vi "Setting.vi"() -> ()   [LabVIEW 2015]
uses:
  enum/Control_PanelControl.ctl
  enum/Control_FileControl.ctl
  enum/Control_ExitControl.ctl
  enum/Control_IOControl.ctl
  enum/Control_CameraControl.ctl
  enum/Control_ImageControl.ctl
  enum/Control_Inspection.ctl
  enum/Control_InspectionItem.ctl
  enum/Control_ErrorControl.ctl
  enum/Control_IdleControl.ctl
  enum/Control_MachineVerification.ctl
  enum/Control_DialogControl.ctl
  enum/Control_LightControl.ctl
  <vilib>/Utility/miscctls.llb/LVPointTypeDef.ctl
  <userlib>/FGV/control/Control_Indicator Action.ctl
  <userlib>/FGV/control/Control_Image.ctl
  <userlib>/FGV/control/Control_Camera.ctl
  <userlib>/FGV/control/Control_Data.ctl
  <vilib>/userdefined/High Color/IMAQdx.ctl
panel:
  in  "start path":path=path "D:/渦輪組裝機參數/Data 資料/Setting Data"
  in  "file (use dialog)":path=path "D:/渦輪組裝機參數/Data 資料/Setting Data"
  out "Image":T1(plugin-control)
  in  "匯入圖片":bool
  out "input cluster":T2
  in  "Control":T3
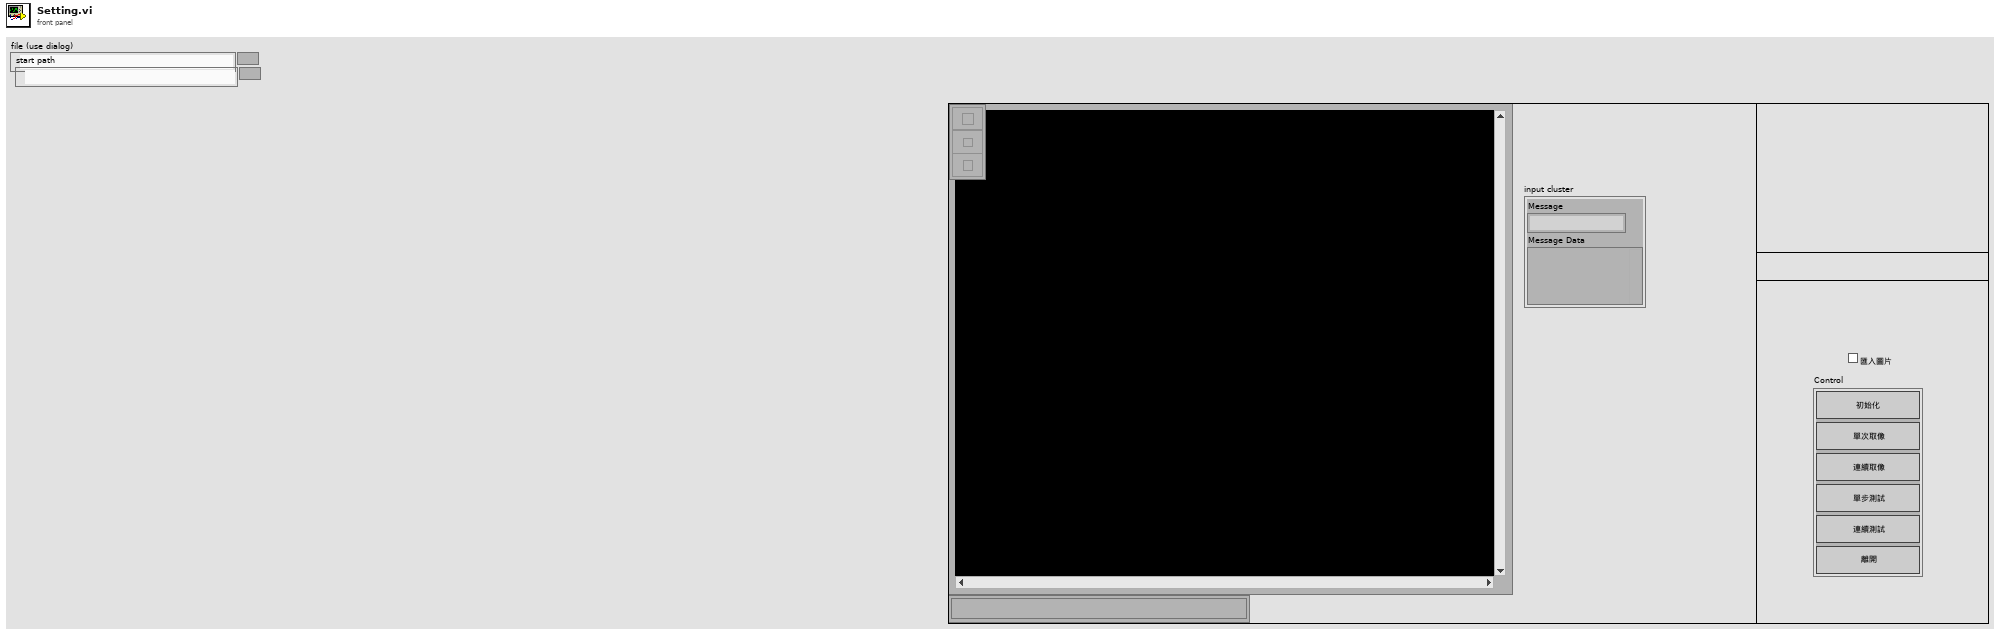
[diagram p1: front panel]
types:
  T1 = typedef "IMAQ Image.ctl" = refnum<image>
  T2 = cluster{"Message":string, "Message Data":variant}
  T3 = cluster{"一、動作-初始化":bool, "二、動作-單次取像":bool, "三、動作-連續取像":bool, "四、動作-單步測試":bool, "五、動作-連續測試":bool, "六、動作-離開":bool}
  T4 = typedef "LVPointTypeDef.ctl" = cluster{"Horizontal":i16, "Vertical":i16}
  T5 = typedef "Control_LightControl.ctl" = enum16{"1.光源控制-初始化", "2.光源控制-光源開啟", "3.光源控制-光源關閉", "4.光源控制-通訊關閉"}
  T6 = typedef "Control_DialogControl.ctl" = enum16{"1.對話視窗"}
  T7 = typedef "Control_MachineVerification.ctl" = enum16{"1.機台驗證-初始化", "2.機台驗證-檢測"}
  T8 = typedef "Control_ExitControl.ctl" = enum16{"1.離開"}
  T9 = typedef "Control_IdleControl.ctl" = enum16{"1.等待(計算時間)"}
  T10 = typedef "Control_ErrorControl.ctl" = enum16{"1.錯誤"}
  T11 = typedef "Control_FileControl.ctl" = enum16{"1.檔案-初始化", "2.檔案-儲存檔案", "3.檔案-開啟檔案", "4.檔案-匯入檔案"}
  T12 = typedef "Control_InspectionItem.ctl" = enum16{"FindPositionXY", "Match"}
  T13 = typedef "Control_Inspection.ctl" = enum16{"1.檢測-初始化", "2.浪代-浪代"}
  T14 = typedef "Control_ImageControl.ctl" = enum16{"1.影像-初始化", "2.影像-更新影像", "3.影像-儲存影像"}
  T15 = typedef "Control_CameraControl.ctl" = enum16{"1.相機-初始化", "2.相機-取像", "3.相機-關閉"}
  T16 = typedef "Control_IOControl.ctl" = enum16{"1.IO-初始化", "2. Set Point(EOT On)", "3.Set Point(EOT Off)", "4.Get Point(SOT)"}
  T17 = typedef "Control_PanelControl.ctl" = enum16{"一、動作-初始化", "二、動作-單次取像", "三、動作-連續取像", "四、動作-單步測試", "五、動作-連續測試", "六、動作-離開"}
  T18 = enum16{"一、動作-初始化", "二、動作-單次取像", "三、動作-連續取像", "四、動作-單步測試", "五、動作-連續測試", "六、動作-離開"}
  T19 = typedef "IMAQdx.ctl" = refnum<k21>
  T20 = typedef "Control_Camera.ctl" = enum16{"初始化", "取像", "匯入影像", "結束"}
  T21 = typedef "Control_Image.ctl" = enum16{"初始化", "創造記憶體", "寫入圖片", "讀取圖片", "刪除圖片", "等待"}
  T22 = typedef "Control_Indicator Action.ctl" = enum16{"Set Data", "Get Data", "Idle"}
  T23 = typedef "Control_Data.ctl" = enum16{"Initialize", "Get Data", "Set Data", "Delete Data", "Idle"}
  T24 = cluster{"Message":string, "Message Data":variant}[]
  T25 = cluster{"Label.Text":string, "Variant":variant}[]
  T26 = typedef "Control_Indicator.ctl" = cluster{"相機、光源":cluster{"相機選擇":u8, "光源選擇":u16, "光源亮度":u8}, "Session Out":T19, "Cam#Light#Strength":string}
  T27 = typedef "Image Type" = u32
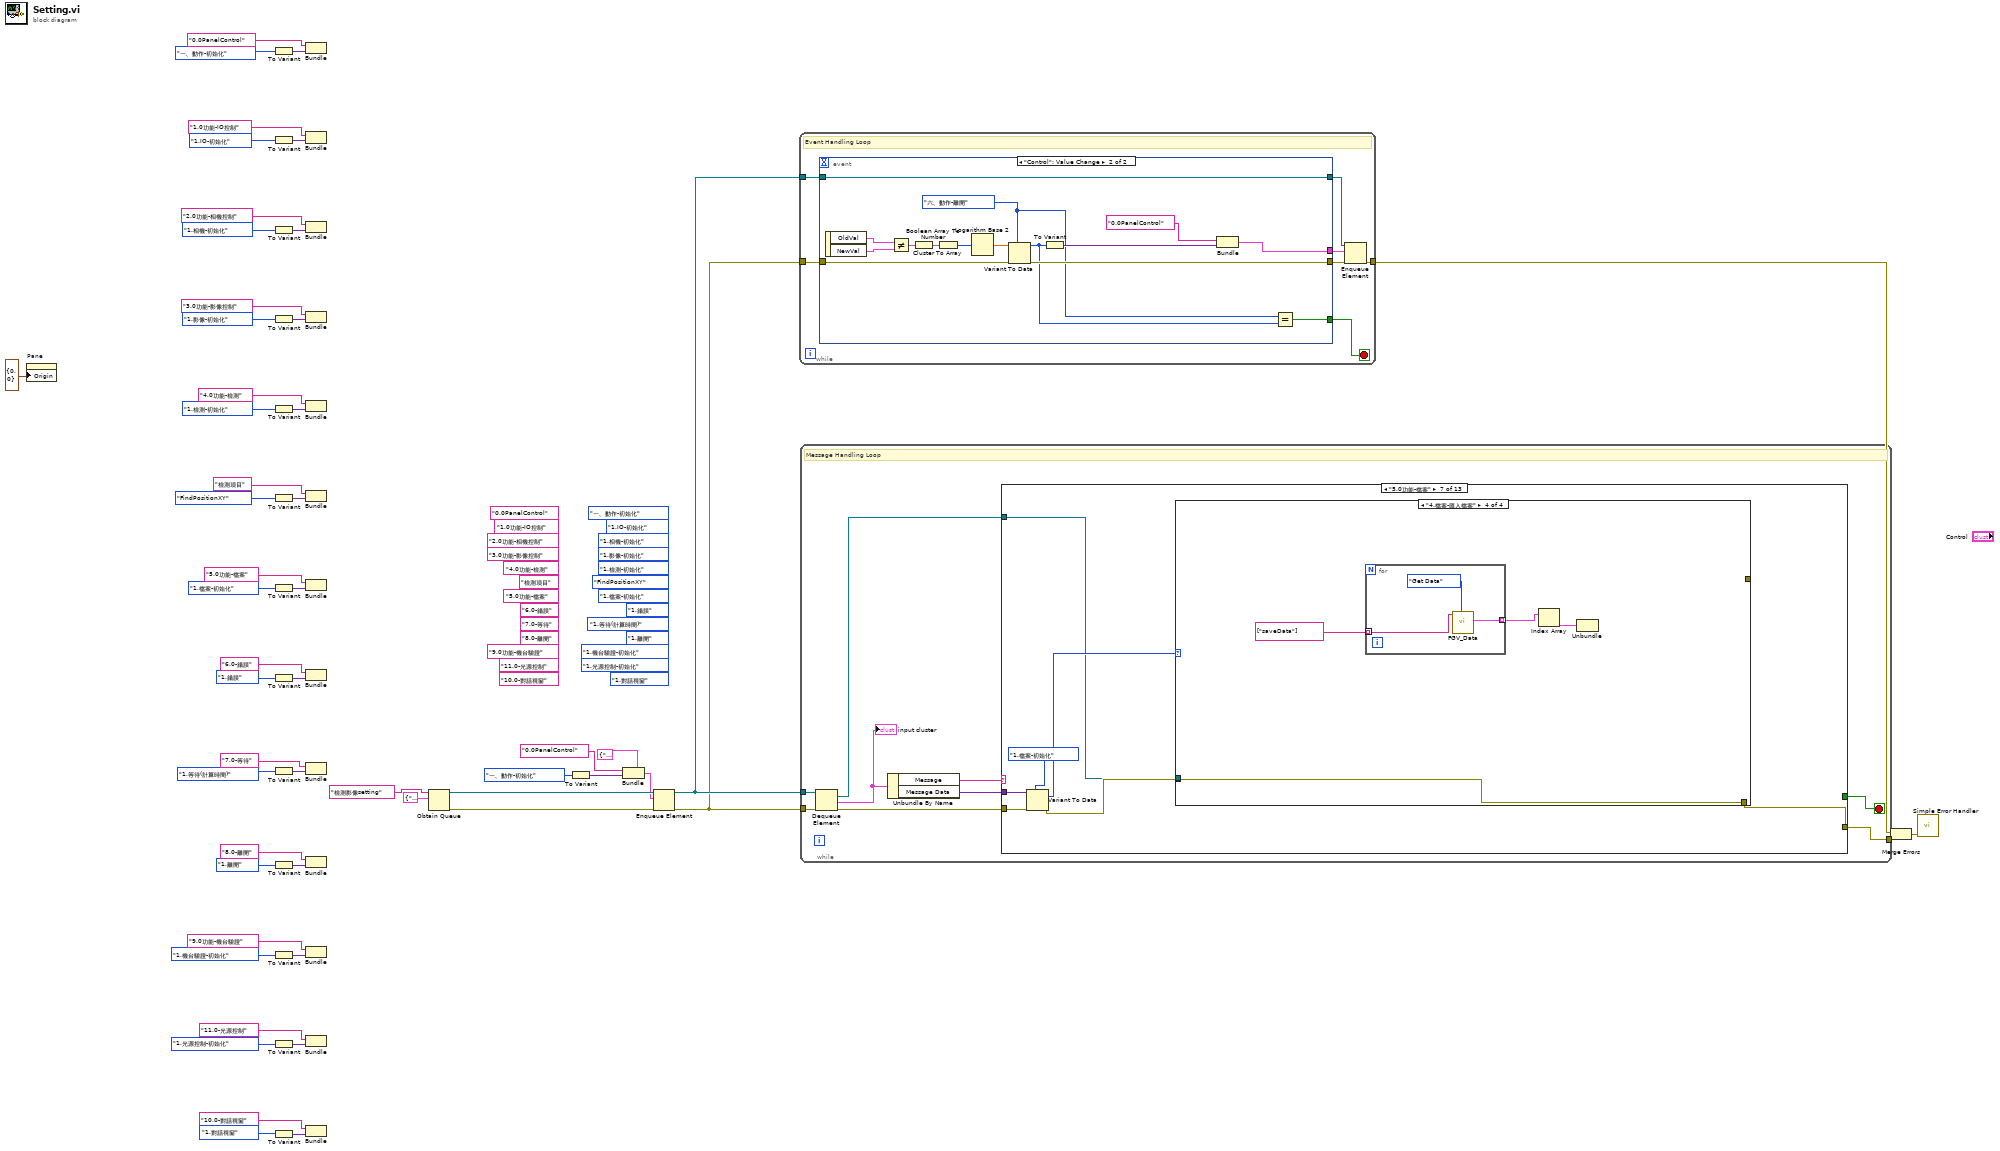
[diagram p0: block diagram]
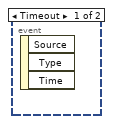
[diagram p2: hidden frame]
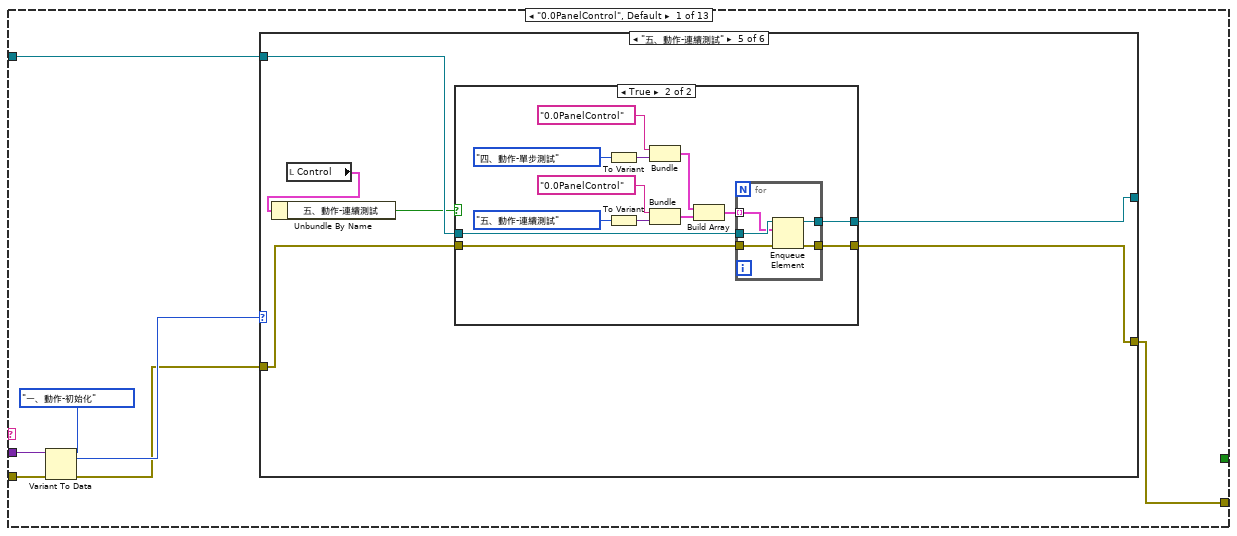
[diagram p3: hidden frame]
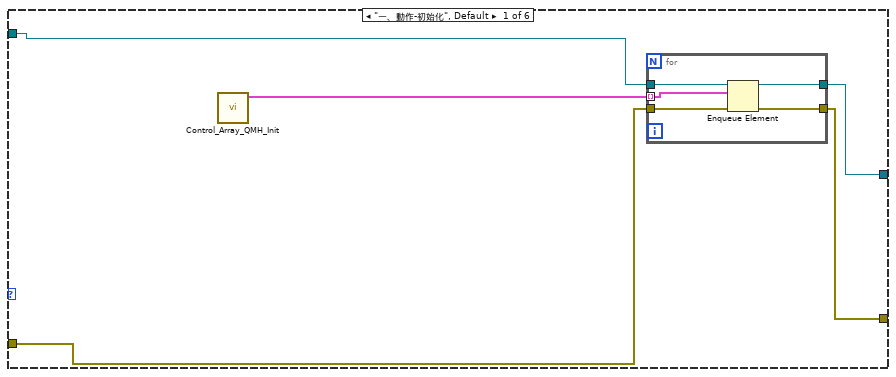
[diagram p4: hidden frame]
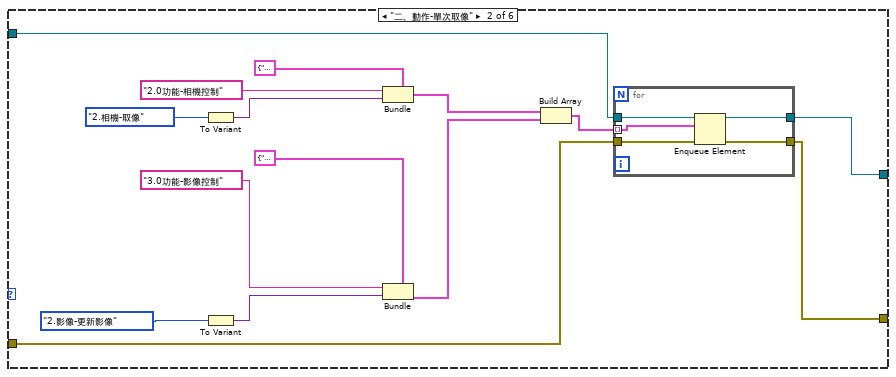
[diagram p5: hidden frame]
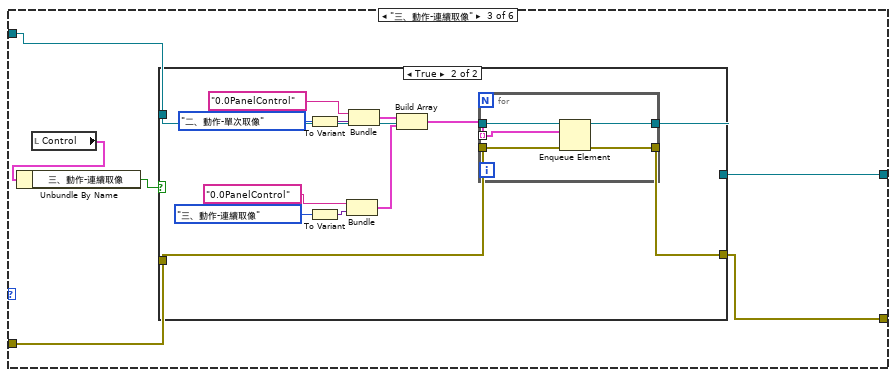
[diagram p6: hidden frame]
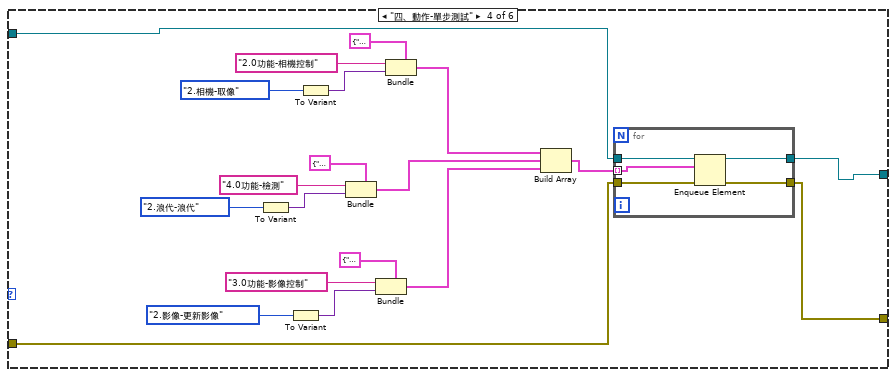
[diagram p8: hidden frame]
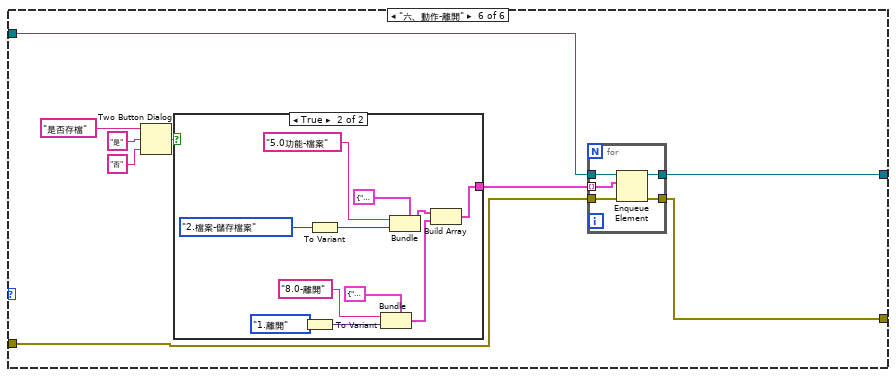
[diagram p10: hidden frame]
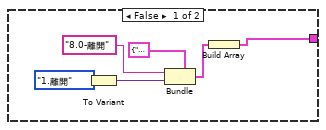
[diagram p11: hidden frame]
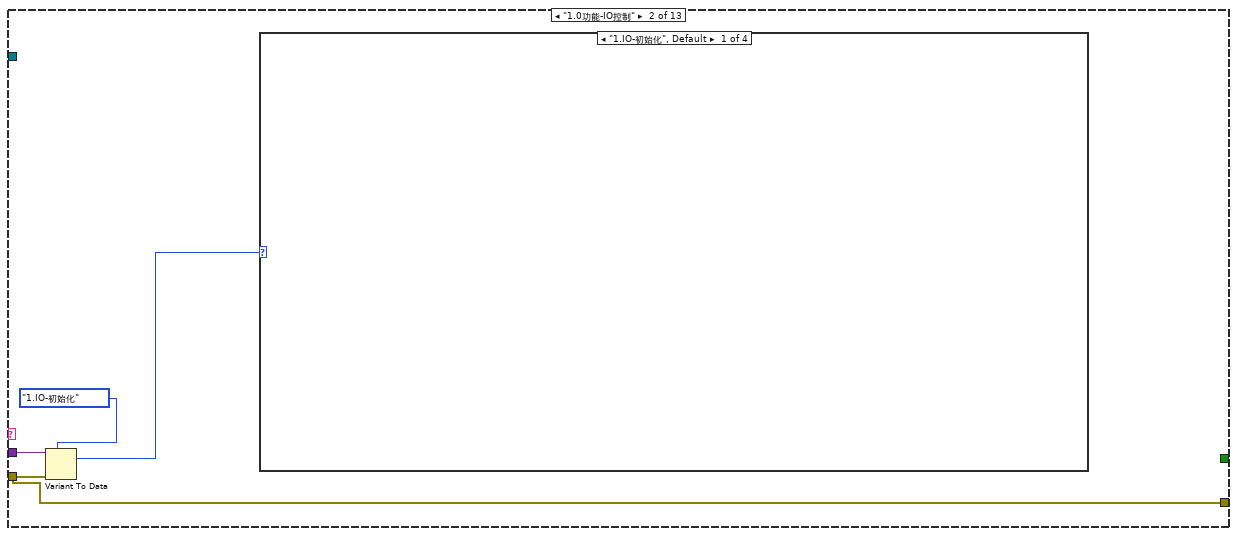
[diagram p12: hidden frame]
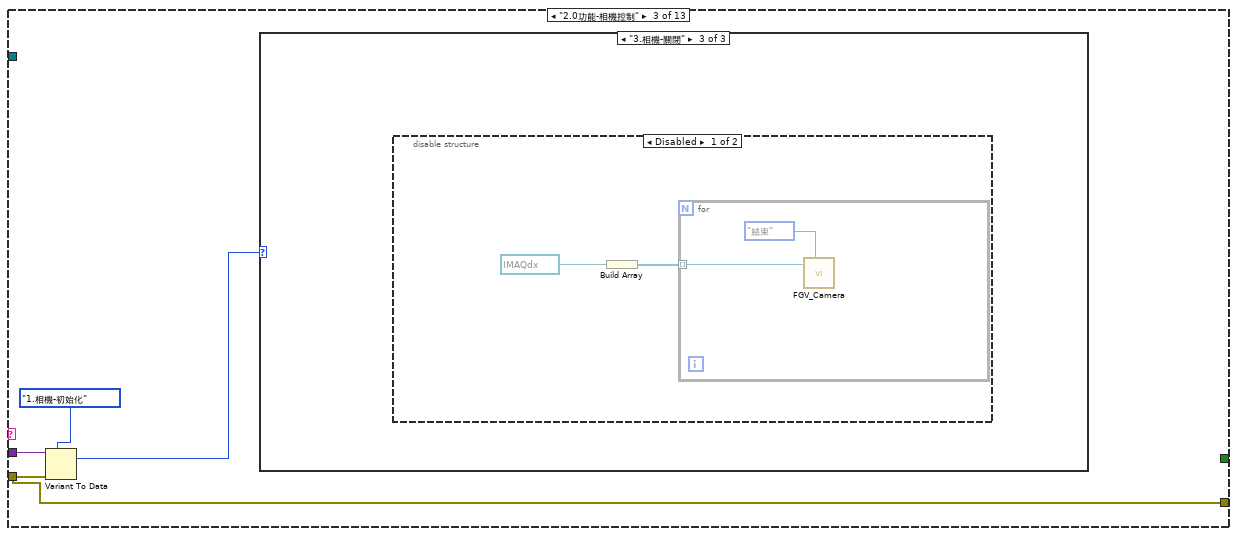
[diagram p16: hidden frame]
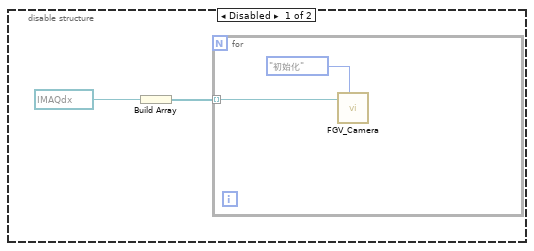
[diagram p18: hidden frame]
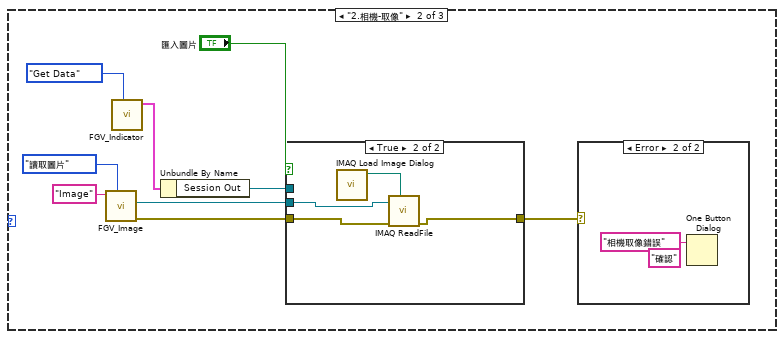
[diagram p19: hidden frame]
diagram:
  (unwired) "11.0-光源控制" ("Label.Text")
  (unwired) "10.0-對話視窗" ("Label.Text")
  (unwired) "9.0功能-機台驗證" ("Label.Text")
  (unwired) "8.0-離開" ("Label.Text")
  (unwired) "7.0-等待" ("Label.Text")
  (unwired) "6.0-錯誤" ("Label.Text")
  (unwired) "5.0功能-檔案" ("Label.Text")
  (unwired) "檢測項目" ("Label.Text")
  (unwired) "4.0功能-檢測" ("Label.Text")
  (unwired) "3.0功能-影像控制" ("Label.Text")
  (unwired) "2.0功能-相機控制" ("Label.Text")
  (unwired) "1.0功能-IO控制" ("Label.Text")
  (unwired) "0.0PanelControl" ("Label.Text")
  (unwired) Control_LightControl."1.光源控制-初始化" ("11.0-光源控制")
  (unwired) Control_DialogControl."1.對話視窗" ("10.0-對話視窗")
  (unwired) Control_MachineVerification."1.機台驗證-初始化" ("9.0功能-機台驗證")
  (unwired) Control_ExitControl."1.離開" ("8.0-離開")
  (unwired) Control_IdleControl."1.等待(計算時間)" ("7.0-等待")
  (unwired) Control_ErrorControl."1.錯誤" ("6.0-錯誤")
  (unwired) Control_FileControl."1.檔案-初始化" ("5.0功能-檔案")
  (unwired) Control_InspectionItem."FindPositionXY" ("檢測項目 2")
  (unwired) Control_Inspection."1.檢測-初始化" ("4.0功能-檢測")
  (unwired) Control_ImageControl."1.影像-初始化" ("3.0功能-影像控制")
  (unwired) Control_CameraControl."1.相機-初始化" ("2.0功能-相機控制")
  (unwired) Control_IOControl."1.IO-初始化" ("1.0 功能-IO控制")
  (unwired) Control_PanelControl."一、動作-初始化" ("0.0PanelControl")
  n1 = property on="Pane" class="Pane"("Origin"=T4 {"Horizontal"=0, "Vertical"=0}) -> ()  [unwired: 2 in, 2 out]
  n2 = To Variant(anything=Control_PanelControl."一、動作-初始化" ("0.0PanelControl")) -> (Variant=w35:variant)
  n3 = To Variant(anything=Control_IOControl."1.IO-初始化" ("1.0 功能-IO控制")) -> (Variant=w23:variant)
  n4 = To Variant(anything=Control_CameraControl."1.相機-初始化" ("2.0功能-相機控制")) -> (Variant=w22:variant)
  n5 = To Variant(anything=Control_ImageControl."1.影像-初始化" ("3.0功能-影像控制")) -> (Variant=w21:variant)
  n6 = To Variant(anything=Control_Inspection."1.檢測-初始化" ("4.0功能-檢測")) -> (Variant=w20:variant)
  n7 = To Variant(anything=Control_InspectionItem."FindPositionXY" ("檢測項目 2")) -> (Variant=w19:variant)
  n8 = To Variant(anything=Control_FileControl."1.檔案-初始化" ("5.0功能-檔案")) -> (Variant=w18:variant)
  n9 = To Variant(anything=Control_ErrorControl."1.錯誤" ("6.0-錯誤")) -> (Variant=w17:variant)
  n10 = To Variant(anything=Control_IdleControl."1.等待(計算時間)" ("7.0-等待")) -> (Variant=w16:variant)
  n11 = To Variant(anything=Control_ExitControl."1.離開" ("8.0-離開")) -> (Variant=w15:variant)
  n12 = To Variant(anything=Control_MachineVerification."1.機台驗證-初始化" ("9.0功能-機台驗證")) -> (Variant=w14:variant)
  n13 = To Variant(anything=Control_LightControl."1.光源控制-初始化" ("11.0-光源控制")) -> (Variant=w12:variant)
  n14 = To Variant(anything=Control_DialogControl."1.對話視窗" ("10.0-對話視窗")) -> (Variant=w13:variant)
  n15 = Bundle("Label.Text"="0.0PanelControl", "Variant"=w35) -> ()  [unwired: 1 in, 1 out]
  n16 = Bundle("Label.Text"="1.0功能-IO控制", "Variant"=w23) -> ()  [unwired: 1 in, 1 out]
  n17 = Bundle("Label.Text"="2.0功能-相機控制", "Variant"=w22) -> ()  [unwired: 1 in, 1 out]
  n18 = Bundle("Label.Text"="3.0功能-影像控制", "Variant"=w21) -> ()  [unwired: 1 in, 1 out]
  n19 = Bundle("Label.Text"="4.0功能-檢測", "Variant"=w20) -> ()  [unwired: 1 in, 1 out]
  n20 = Bundle("Label.Text"="檢測項目", "Variant"=w19) -> ()  [unwired: 1 in, 1 out]
  n21 = Bundle("Label.Text"="5.0功能-檔案", "Variant"=w18) -> ()  [unwired: 1 in, 1 out]
  n22 = Bundle("Label.Text"="6.0-錯誤", "Variant"=w17) -> ()  [unwired: 1 in, 1 out]
  n23 = Bundle("Label.Text"="7.0-等待", "Variant"=w16) -> ()  [unwired: 1 in, 1 out]
  n24 = Bundle("Label.Text"="8.0-離開", "Variant"=w15) -> ()  [unwired: 1 in, 1 out]
  n25 = Bundle("Label.Text"="9.0功能-機台驗證", "Variant"=w14) -> ()  [unwired: 1 in, 1 out]
  n26 = Bundle("Label.Text"="11.0-光源控制", "Variant"=w12) -> ()  [unwired: 1 in, 1 out]
  n27 = Bundle("Label.Text"="10.0-對話視窗", "Variant"=w13) -> ()  [unwired: 1 in, 1 out]
  n28 = Obtain Queue(name (unnamed)="檢測影像setting", element data type=T2 {"Message"="", "Message Data"=variant} ("element")) -> (queue out=w52:refnum<queue>, error out=w53:errorcluster)  [unwired: 3 in, 1 out]
  n29 = To Variant(anything=Control_PanelControl."一、動作-初始化" ("0.0PanelControl 2")) -> (Variant=w8:variant)
  n30 = Bundle(cluster=T2 {"Message"="", "Message Data"=variant} ("element"), "Message"="0.0PanelControl" ("Label.Text"), "Message Data"=w8) -> (w7:T2)
  n31 = Enqueue Element(queue=w52, element=w7, error in (no error)=w53) -> (queue out=w51:refnum<queue>, error out=w4:errorcluster)  [unwired: 1 in, 1 out]
  n32 = while {
    tunnel: w51 -> [w55]
    tunnel: w4 -> [w61]
    tunnel: [w58] -> w3
    stop <- w57 stop-if-true
    # "Event Handling Loop"
    n33 = event shown="[1] \"Control\": Value Change" {
      selector: _ -> [_ _]
      dyn-events: _ -> [_ _]
      timeout: _ -> [_ _]
      tunnel: w61 -> [_ w68]
      tunnel: [_ w67] -> w60
      tunnel: [_ w66] -> w59
      tunnel: [_ w63] -> w57
      tunnel: [_ w62] -> w56
      tunnel: w55 -> [_ w62]
      event Timeout {
        n34 = event-data() -> ()  [unwired: 1 in, 3 out]
      }
      event "Control": Value Change {
        w65 = T18."六、動作-離開" ("0.0PanelControl")
        n35 = event-data() -> ("OldVal"=w70:T3, "NewVal"=w69:T3)  [unwired: 1 in]
        n36 = Not Equal?(x=w70, y=w69) -> (x != y?=w76:T3)
        n37 = Cluster To Array(cluster=w76) -> (array=w75:bool[])
        n38 = Boolean Array To Number(Boolean array=w75) -> (number=w74:u32)
        n39 = Logarithm Base 2(1:w74) -> (0:w73:dbl)
        n40 = Variant To Data(error in=w68, type=w65, Variant=w73) -> (data=w64:T18, error out=w67:errorcluster)
        n41 = To Variant(anything=w64) -> (Variant=w71:variant)
        n42 = Bundle("0.0PanelControl", "Variant"=w71) -> (w66:cluster{string, "Variant":variant})  [unwired: 1 in]
        n43 = Equal?(x=w65, y=w64) -> (x = y?=w63:bool)
      }
    }
    n44 = Enqueue Element(queue=w56, element=w59, error in (no error)=w60) -> (error out=w58:errorcluster)  [unwired: 1 in, 2 out]
  }
  n45 = while {
    tunnel: w51 -> [w84]
    tunnel: w4 -> [w85]
    tunnel: [w82] -> w54
    stop <- w80 stop-if-true
    # "Message Handling Loop"
    n46 = Dequeue Element(queue=w84, error in (no error)=w85) -> (queue out=w81:refnum<queue>, element=w79:T2, error out=w83:errorcluster)  [unwired: 1 in, 1 out]
    "input cluster" <- w79
    n47 = Unbundle By Name(w79) -> ("Message"=w78:string, "Message Data"=w77:variant)
    n48 = case shown="\"5.0功能-檔案\"" w78 {
      tunnel: w83 -> [w89 w231 w235 w271 w288 w292 w298 w340 w344 w349 w354 w358 w362]
      tunnel: [w87 w231 w235 w271 w288 w292 w297 w340 w344 w349 w354 w358 w362] -> w82
      tunnel: w81 -> [w90 _ _ _ _ _ w296 _ _ _ _ _ _]
      tunnel: w77 -> [w92 w234 w237 w274 w291 w295 w302 w343 w347 w352 w357 w361 w365]
      tunnel: [_ _ _ _ _ _ _ _ _ w348 _ _ _] -> w80
      frame "0.0PanelControl", Default {
        n49 = Variant To Data(error in=w89, type=Control_PanelControl."一、動作-初始化" ("0.0PanelControl"), Variant=w92) -> (data=w91:T17, error out=w88:errorcluster)
        n50 = case shown="\"五、動作-連續測試\"" w91 {
          tunnel: w90 -> [w96 w105 w128 w153 w179 w203]
          tunnel: w88 -> [w97 w104 w127 w152 w178 w202]
          tunnel: [w94 w117 w126 w151 w177 w201] -> w87
          tunnel: [w93 w103 w125 w149 w176 w200] -> _
          frame "一、動作-初始化", Default {
            n51 = call "Control_Array_QMH_Init.vi"() -> ("Init setting"=w95:T24)  [unwired: 11 in]
            n52 = for {
              tunnel: w96 -> [w102]
              tunnel: w97 -> [w101]
              tunnel: [w100] -> w94
              tunnel: [w99] -> w93
              tunnel: w95 -> [w98] mode=indexing
              n53 = Enqueue Element(queue=w102, element=w98, error in (no error)=w101) -> (queue out=w99:refnum<queue>, error out=w100:errorcluster)  [unwired: 1 in, 1 out]
            }
          }
          frame "二、動作-單次取像" {
            n54 = To Variant(anything=Control_CameraControl."2.相機-取像" ("2.0功能-相機控制")) -> (Variant=w110:variant)
            n55 = To Variant(anything=Control_ImageControl."2.影像-更新影像" ("3.0功能-影像控制")) -> (Variant=w109:variant)
            n56 = Bundle(cluster=T2 {"Message"="", "Message Data"=variant} ("element"), "Message"="2.0功能-相機控制" ("Label.Text"), "Message Data"=w110) -> (w108:T2)
            n57 = Bundle(cluster=T2 {"Message"="", "Message Data"=variant} ("element"), "Message"="3.0功能-影像控制" ("Label.Text"), "Message Data"=w109) -> (w107:T2)
            n58 = Build Array(w108, w107) -> (w106:T24)
            n59 = for {
              tunnel: w105 -> [w122]
              tunnel: w104 -> [w121]
              tunnel: [w120] -> w117
              tunnel: [w119] -> w103
              tunnel: w106 -> [w118] mode=indexing
              n60 = Enqueue Element(queue=w122, element=w118, error in (no error)=w121) -> (queue out=w119:refnum<queue>, error out=w120:errorcluster)  [unwired: 1 in, 1 out]
            }
          }
          frame "三、動作-連續取像" {
            n61 = local read "Control"() -> (w124:T3)
            n62 = Unbundle By Name(w124) -> ("三、動作-連續取像"=w123:bool)
            n63 = case shown="True" w123 {
              tunnel: w128 -> [w130 w142]
              tunnel: w127 -> [w129 w141]
              tunnel: [w129 w140] -> w126
              tunnel: [w130 w131] -> w125
              frame False {
              }
              frame True {
                n64 = To Variant(anything=Control_PanelControl."二、動作-單次取像" ("0.0PanelControl")) -> (Variant=w137:variant)
                n65 = To Variant(anything=Control_PanelControl."三、動作-連續取像" ("0.0PanelControl")) -> (Variant=w135:variant)
                n66 = Bundle("Label.Text"="0.0PanelControl", "Variant"=w135) -> (w132:cluster{"Label.Text":string, "Variant":variant})  [unwired: 1 in]
                n67 = Bundle("Label.Text"="0.0PanelControl", "Variant"=w137) -> (w136:cluster{"Label.Text":string, "Variant":variant})  [unwired: 1 in]
                n68 = Build Array(w136, w132) -> (w143:T25)
                n69 = for {
                  tunnel: w142 -> [w148]
                  tunnel: w141 -> [w147]
                  tunnel: [w146] -> w140
                  tunnel: [w145] -> w131
                  tunnel: w143 -> [w144] mode=indexing
                  n70 = Enqueue Element(queue=w148, element=w144, error in (no error)=w147) -> (queue out=w145:refnum<queue>, error out=w146:errorcluster)  [unwired: 1 in, 1 out]
                }
              }
            }
          }
          frame "四、動作-單步測試" {
            n71 = To Variant(anything=Control_Inspection."2.浪代-浪代" ("4.0功能-檢測")) -> (Variant=w157:variant)
            n72 = To Variant(anything=Control_ImageControl."2.影像-更新影像" ("3.0功能-影像控制")) -> (Variant=w158:variant)
            n73 = To Variant(anything=Control_CameraControl."2.相機-取像" ("2.0功能-相機控制")) -> (Variant=w159:variant)
            n74 = Bundle(cluster=T2 {"Message"="", "Message Data"=variant} ("element"), "Message"="4.0功能-檢測" ("Label.Text"), "Message Data"=w157) -> (w154:T2)
            n75 = Bundle(cluster=T2 {"Message"="", "Message Data"=variant} ("element"), "Message"="3.0功能-影像控制" ("Label.Text"), "Message Data"=w158) -> (w155:T2)
            n76 = Bundle(cluster=T2 {"Message"="", "Message Data"=variant} ("element"), "Message"="2.0功能-相機控制" ("Label.Text"), "Message Data"=w159) -> (w156:T2)
            n77 = Build Array(w156, w154, w155) -> (w150:T24)
            n78 = for {
              tunnel: w153 -> [w173]
              tunnel: w152 -> [w172]
              tunnel: [w171] -> w151
              tunnel: [w170] -> w149
              tunnel: w150 -> [w169] mode=indexing
              n79 = Enqueue Element(queue=w173, element=w169, error in (no error)=w172) -> (queue out=w170:refnum<queue>, error out=w171:errorcluster)  [unwired: 1 in, 1 out]
            }
          }
          frame "五、動作-連續測試" {
            n80 = local read "Control"() -> (w175:T3)
            n81 = Unbundle By Name(w175) -> ("五、動作-連續測試"=w174:bool)
            n82 = case shown="True" w174 {
              tunnel: w179 -> [w181 w185]
              tunnel: w178 -> [w180 w184]
              tunnel: [w180 w183] -> w177
              tunnel: [w181 w182] -> w176
              frame False {
              }
              frame True {
                n83 = To Variant(anything=Control_PanelControl."四、動作-單步測試" ("0.0PanelControl")) -> (Variant=w191:variant)
                n84 = To Variant(anything=Control_PanelControl."五、動作-連續測試" ("0.0PanelControl")) -> (Variant=w189:variant)
                n85 = Bundle("Label.Text"="0.0PanelControl", "Variant"=w191) -> (w190:cluster{"Label.Text":string, "Variant":variant})  [unwired: 1 in]
                n86 = Bundle("Label.Text"="0.0PanelControl", "Variant"=w189) -> (w186:cluster{"Label.Text":string, "Variant":variant})  [unwired: 1 in]
                n87 = Build Array(w190, w186) -> (w194:T25)
                n88 = for {
                  tunnel: w185 -> [w199]
                  tunnel: w184 -> [w198]
                  tunnel: [w197] -> w183
                  tunnel: [w196] -> w182
                  tunnel: w194 -> [w195] mode=indexing
                  n89 = Enqueue Element(queue=w199, element=w195, error in (no error)=w198) -> (queue out=w196:refnum<queue>, error out=w197:errorcluster)  [unwired: 1 in, 1 out]
                }
              }
            }
          }
          frame "六、動作-離開" {
            n90 = Two Button Dialog(message="是否存檔", 1:"否" ("F button name (\"Cancel\")"), 2:"是" ("T button name (\"OK\")")) -> (T button?=w208:bool)
            n91 = case shown="True" w208 {
              tunnel: [w214 w215] -> w204
              frame False {
                n92 = To Variant(anything=Control_ExitControl."1.離開" ("8.0-離開")) -> (Variant=w213:variant)
                n93 = Bundle(cluster=T2 {"Message"="", "Message Data"=variant} ("element"), "Message"="8.0-離開" ("Label.Text"), "Message Data"=w213) -> (w209:T2)
                n94 = Build Array(w209) -> (w214:T24)
              }
              frame True {
                n95 = To Variant(anything=Control_ExitControl."1.離開" ("8.0-離開")) -> (Variant=w225:variant)
                n96 = To Variant(anything=Control_FileControl."2.檔案-儲存檔案" ("5.0功能-檔案")) -> (Variant=w224:variant)
                n97 = Bundle(cluster=T2 {"Message"="", "Message Data"=variant} ("element"), "Message"="8.0-離開" ("Label.Text"), "Message Data"=w225) -> (w217:T2)
                n98 = Bundle(cluster=T2 {"Message"="", "Message Data"=variant} ("element"), "Message"="5.0功能-檔案" ("Label.Text"), "Message Data"=w224) -> (w216:T2)
                n99 = Build Array(w216, w217) -> (w215:T24)
              }
            }
            n100 = for {
              tunnel: w203 -> [w230]
              tunnel: w202 -> [w229]
              tunnel: [w228] -> w200
              tunnel: [w227] -> w201
              tunnel: w204 -> [w226] mode=indexing
              n101 = Enqueue Element(queue=w230, element=w226, error in (no error)=w229) -> (queue out=w228:refnum<queue>, error out=w227:errorcluster)  [unwired: 1 in, 1 out]
            }
          }
        }
      }
      frame "1.0功能-IO控制" {
        n102 = Variant To Data(error in=w231, type=Control_IOControl."1.IO-初始化" ("1.0 功能-IO控制"), Variant=w234) -> (data=w232:T16)  [unwired: 1 out]
        n103 = case shown="\"1.IO-初始化\", Default" w232 {
          frame "1.IO-初始化", Default {
          }
          frame "2. Set Point(EOT On)" {
          }
          frame "3.Set Point(EOT Off)" {
          }
          frame "4.Get Point(SOT)" {
          }
        }
      }
      frame "2.0功能-相機控制" {
        n104 = Variant To Data(error in=w235, type=Control_CameraControl."1.相機-初始化" ("2.0功能-相機控制"), Variant=w237) -> (data=w236:T15)  [unwired: 1 out]
        n105 = case shown="\"3.相機-關閉\"" w236 {
          frame "1.相機-初始化", Default {
            n106 = disable-structure shown="Enabled" {
              frame Disabled {
                n107 = Build Array(T19 "cam0" ("Session In")) -> (w239:T19[])
                n108 = for {
                  tunnel: w239 -> [w242] mode=indexing
                  n109 = call <userlib>:"FGV_Camera.vi"("action_camera"=Control_Camera."初始化", "Session In"=w242) -> ()  [unwired: 7 in, 3 out]
                }
              }
              frame Enabled {
              }
            }
          }
          frame "2.相機-取像" {
            n110 = call <userlib>:"FGV_Image.vi"("Image action"=Control_Image."讀取圖片", "圖片名稱"="Image") -> ("error out"=w243:errorcluster, "Image Out"=w245:T1)  [unwired: 8 in]
            n111 = call <userlib>:"FGV_Indicator.vi"("Action"=Control_Indicator_Action."Get Data") -> ("Indicator Data Out"=w248:T26)  [unwired: 10 in]
            n112 = Unbundle By Name(w248) -> ("Session Out"=w246:T19)
            n113 = case shown="True" "匯入圖片" {
              tunnel: w246 -> [w260 _]
              tunnel: w245 -> [w259 w262]
              tunnel: [w254 w264] -> w244
              tunnel: w243 -> [w253 w263]
              frame False {
                n114 = call <userlib>:"FGV_Camera.vi"("action_camera"=Control_Camera."取像", "error in"=w253, "Image In"=w259, "Session In"=w260) -> ("error out"=w255:errorcluster, "Image Out"=w256:T1)  [unwired: 5 in, 1 out]
                n115 = call <userlib>:"FGV_Image.vi"("Image action"=Control_Image."寫入圖片", "error in (no error)"=w255, "Image In"=w256, "圖片名稱"="Image") -> ("error out"=w254:errorcluster)  [unwired: 6 in, 1 out]
              }
              frame True {
                n116 = call "IMAQ Load Image Dialog"() -> ("Path"=w265:path)  [unwired: 9 in, 2 out]
                n117 = call "IMAQ ReadFile"("File Path"=w265, "error in (no error)"=w263, "Image"=w262) -> ("error out"=w264:errorcluster)  [unwired: 4 in, 4 out]
              }
            }
            n118 = case shown="Error" w244 {
              frame No Error {
              }
              frame Error {
                (unwired) "確認" ("button name (\"OK\")")
                n119 = One Button Dialog(message="相機取像錯誤") -> ()  [unwired: 1 in, 1 out]
              }
            }
          }
          frame "3.相機-關閉" {
            n120 = disable-structure shown="Disabled" {
              frame Disabled {
                n121 = Build Array(T19 "cam0" ("Session In")) -> (w266:T19[])
                n122 = for {
                  tunnel: w266 -> [w269] mode=indexing
                  n123 = call <userlib>:"FGV_Camera.vi"("action_camera"=Control_Camera."結束", "Session In"=w269) -> ()  [unwired: 7 in, 3 out]
                }
              }
              frame Enabled {
              }
            }
          }
        }
      }
      frame "3.0功能-影像控制" {
        n124 = Variant To Data(error in=w271, type=Control_ImageControl."1.影像-初始化" ("3.0功能-影像控制"), Variant=w274) -> (data=w272:T14, error out=w270:errorcluster)
        n125 = case shown="\"1.影像-初始化\", Default" w272 {
          tunnel: w270 -> [w275 w284 _]
          frame "1.影像-初始化", Default {
            n126 = disable-structure shown="Enabled" {
              disable-tunnel: w275 -> [w279 _]
              frame Enabled {
                w277 = T27[] [0] items=["Grayscale (U8)", "Grayscale (I16)", "Grayscale (SGL)", "Complex (CSG)", "RGB (U32)", "HSL (U32)", "RGB (U64)", "Grayscale (U16)"]
                n127 = call <userlib>:"FGV_Image.vi"("error in (no error)"=w279) -> ("error out"=w276:errorcluster)  [unwired: 9 in, 1 out]
                n128 = for {
                  tunnel: string[] ["Image"] -> [w282] mode=indexing
                  tunnel: w277 -> [w281] mode=indexing
                  tunnel: w276 -> [w280]
                  n129 = call <userlib>:"FGV_Image.vi"("Image action"=Control_Image."創造記憶體", "error in (no error)"=w280, "Image Type"=w281, "圖片名稱"=w282) -> ()  [unwired: 6 in, 2 out]
                }
              }
              frame Disabled {
              }
            }
          }
          frame "2.影像-更新影像" {
            n130 = call <userlib>:"FGV_Image.vi"("Image action"=Control_Image."讀取圖片", "error in (no error)"=w284, "圖片名稱"="Image") -> ("Image Out"=→"Image":T1)  [unwired: 7 in, 1 out]
          }
          frame "3.影像-儲存影像" {
          }
        }
      }
      frame "4.0功能-檢測" {
        n131 = Variant To Data(error in=w288, type=Control_Inspection."1.檢測-初始化" ("4.0功能-檢測"), Variant=w291) -> (data=w289:T13)  [unwired: 1 out]
        n132 = case shown="\"1.檢測-初始化\", Default" w289 {
          frame "1.檢測-初始化", Default {
          }
          frame "2.浪代-浪代" {
          }
        }
      }
      frame "檢測項目" {
        n133 = Variant To Data(error in=w292, type=Control_InspectionItem."FindPositionXY" ("檢測項目 2"), Variant=w295) -> (data=w293:T12)  [unwired: 1 out]
        n134 = case shown="\"FindPositionXY\", Default" w293 {
          frame "FindPositionXY", Default {
          }
          frame "Match" {
          }
        }
      }
      frame "5.0功能-檔案" {
        n135 = Variant To Data(error in=w298, type=Control_FileControl."1.檔案-初始化" ("5.0功能-檔案"), Variant=w302) -> (data=w300:T11, error out=w299:errorcluster)
        n136 = case shown="\"4.檔案-匯入檔案\"" w300 {
          tunnel: w299 -> [w304 w309 w329 w336]
          tunnel: [w303 w309 w329 w336] -> w297
          tunnel: w296 -> [_ _ w328 _]
          tunnel: [_ _ w317 _] -> _
          frame "1.檔案-初始化", Default {
            n137 = call <userlib>:"FGV_Data.vi"("Action_Data"=Control_Data."Initialize", "error in"=w304) -> ("error out"=w303:errorcluster)  [unwired: 7 in, 2 out]
          }
          frame "2.檔案-儲存檔案" {
            n138 = call <userlib>:"FGV_Indicator.vi"("Action"=Control_Indicator_Action."Get Data") -> ("Indicator Data Out"=w314:T26)  [unwired: 10 in]
            n139 = Unbundle By Name(w314) -> ("相機、光源.相機選擇"=w313:u8)
            n140 = call <userlib>:"FGV_Data.vi"("Action_Data"=Control_Data."Idle") -> ("Data Array out"=w308:cluster{"Data name":string, "Data":variant}[])  [unwired: 8 in, 2 out]
            n141 = case shown="0, Default" w313 {
              tunnel: ["CCD1"] -> w306
              frame 0, Default {
              }
            }
            n142 = Build Path(base path="file (use dialog)", name or relative path=w306) -> (appended path=w311:path)
            n143 = Build Path(base path=w311, name or relative path=w306) -> (appended path=w307:path)
            n144 = Write to Binary File(file (use dialog)=w307, data=w308) -> ()  [unwired: 4 in, 3 out]
          }
          frame "3.檔案-開啟檔案" {
            n145 = call "File Dialog"("start path"="start path") -> ("selected path"=w321:path, "error out"=w318:errorcluster)  [unwired: 11 in, 2 out]
            n146 = Read from Binary File(5:cluster{"Data name":string, "Data":variant}[] [] ("Data Array out"), 8:w318, 11:w321) -> (0:w317:errorcluster, 2:w319:cluster{"Data name":string, "Data":variant}[])  [unwired: 3 in, 2 out]
            n147 = for {
              tunnel: w319 -> [w330] mode=indexing
              n148 = Unbundle(w330) -> ("Data name"=w332:string)  [unwired: 1 out]
              n149 = call <userlib>:"FGV_Data.vi"("Action_Data"=Control_Data."Set Data", "Data In"=w330, "Data name"=w332) -> ()  [unwired: 6 in, 3 out]
            }
            n150 = To Variant(anything=Control_ImageControl."1.影像-初始化" ("3.0功能-影像控制")) -> (Variant=w324:variant)
            n151 = Bundle(cluster=T2 {"Message"="", "Message Data"=variant} ("element"), "Message"="3.0功能-影像控制" ("Label.Text"), "Message Data"=w324) -> (w323:T2)
            n152 = Enqueue Element(queue=w328, element=w323) -> ()  [unwired: 2 in, 3 out]
          }
          frame "4.檔案-匯入檔案" {
            n153 = for {
              tunnel: string[] ["saveData"] -> [w339] mode=indexing
              tunnel: [w337] -> w334 mode=indexing
              n154 = call <userlib>:"FGV_Data.vi"("Action_Data"=Control_Data."Get Data", "Data name"=w339) -> ("Data  Out"=w337:cluster{"Data name":string, "Data":variant})  [unwired: 7 in, 2 out]
            }
            n155 = Index Array(array=w334) -> (element=w333:cluster{"Data name":string, "Data":variant})  [unwired: 1 in]
            n156 = Unbundle(w333) -> ()  [unwired: 2 out]
          }
        }
      }
      frame "6.0-錯誤" {
        n157 = Variant To Data(error in=w340, type=Control_ErrorControl."1.錯誤" ("6.0-錯誤"), Variant=w343) -> (data=w341:T10)  [unwired: 1 out]
        n158 = case shown="\"1.錯誤\", Default" w341 {
          frame "1.錯誤", Default {
          }
        }
      }
      frame "7.0-等待" {
        n159 = Variant To Data(error in=w344, type=Control_IdleControl."1.等待(計算時間)" ("7.0-等待"), Variant=w347) -> (data=w345:T9)  [unwired: 1 out]
        n160 = case shown="\"1.等待(計算時間)\", Default" w345 {
          frame "1.等待(計算時間)", Default {
          }
        }
      }
      frame "8.0-離開" {
        n161 = Variant To Data(error in=w349, type=Control_ExitControl."1.離開" ("8.0-離開"), Variant=w352) -> (data=w350:T8)  [unwired: 1 out]
        n162 = case shown="\"1.離開\", Default" w350 {
          tunnel: [TRUE] -> w348
          frame "1.離開", Default {
          }
        }
      }
      frame "9.0功能-機台驗證" {
        n163 = Variant To Data(error in=w354, type=Control_MachineVerification."1.機台驗證-初始化" ("9.0功能-機台驗證"), Variant=w357) -> (data=w355:T7)  [unwired: 1 out]
        n164 = case shown="\"1.機台驗證-初始化\", Default" w355 {
          frame "1.機台驗證-初始化", Default {
          }
          frame "2.機台驗證-檢測" {
          }
        }
      }
      frame "10.0-對話視窗" {
        n165 = Variant To Data(error in=w358, type=Control_DialogControl."1.對話視窗" ("10.0-對話視窗"), Variant=w361) -> (data=w359:T6)  [unwired: 1 out]
        n166 = case shown="\"1.對話視窗\", Default" w359 {
          frame "1.對話視窗", Default {
          }
        }
      }
      frame "11.0-光源控制" {
        n167 = Variant To Data(error in=w362, type=Control_LightControl."1.光源控制-初始化" ("11.0-光源控制"), Variant=w365) -> (data=w363:T5)  [unwired: 1 out]
        n168 = case shown="\"3.光源控制-光源關閉\"" w363 {
          frame "1.光源控制-初始化", Default {
          }
          frame "2.光源控制-光源開啟" {
          }
          frame "3.光源控制-光源關閉" {
          }
          frame "4.光源控制-通訊關閉" {
          }
        }
      }
    }
  }
  n169 = Merge Errors(w3, w54) -> (w50:errorcluster)
  n170 = call <vilib>:"Simple Error Handler.vi"("error in (no error)"=w50) -> ()  [unwired: 4 in, 5 out]
